vi "host.vi"() -> ()   [LabVIEW 2020]
uses:
  <vilib>/Analysis/baseanly.llb/Real A x B.vi
  <vilib>/Analysis/baseanly.llb/Mean (DBL).vi
  <vilib>/Analysis/Matrix/Numeric/Conversions/Array To Matrix - RA2.vi
  <vilib>/Analysis/Matrix/Numeric/Conversions/Matrix To Array - RM.vi
  <vilib>/Analysis/7linalg.llb/Real Eigenvalues and Vectors.vi
  <vilib>/FPGAPlugInAG/cRIO-9035/niLvFpga_Open_cRIO-9035.vi
  <vilib>/rvi/interface/common/dynamic/niFpgaDynamicAddResources.vi
  <vilib>/Utility/error.llb/Error Cluster From Error Code.vi
  <vilib>/rvi/errors/niLvFpgaAdjustHostInterfaceError.vi
  <vilib>/FPGAPlugInAG/Dynamic/niLvFpga_Run_Dynamic.vi
  <vilib>/FPGAPlugInAG/Dynamic/niLvFpga_Close_Dynamic.vi
  <vilib>/rvi/interface/nirviOpenFPGA/nirviOpenFPGA.xnode
  FPGA Bitfiles/v1.1_FPGATarget_target_IynmV97gzEU.lvbitx
  target.vi
  <vilib>/rvi/interface/nirviMethod/nirviMethod.xnode
  <vilib>/rvi/interface/nirviCloseFPGA/nirviCloseFPGA.xnode
  <vilib>/rvi/errors/niLvFpgaMergeErrorWithErrorCode.vi
  <vilib>/Analysis/Matrix/NI_Matrix.lvlib
  <vilib>/Analysis/NI_AALBase.lvlib
  <vilib>/FPGAPlugInAG/Dynamic/niLvFpga_WriteFifo_Dynamic.vi
  <vilib>/FPGAPlugInAG/Dynamic/niLvFpga_ReadFifo_Dynamic.vi
  <vilib>/Analysis/NI_AALPro.lvlib
panel:
  out "A":dbl[][](array[numeric])
  out "LabVIEW eigvals":dbl[](array[numeric])
  out "FPGA Jacobi eigenvalue":sgl[](array[numeric])
  out "percent error":dbl
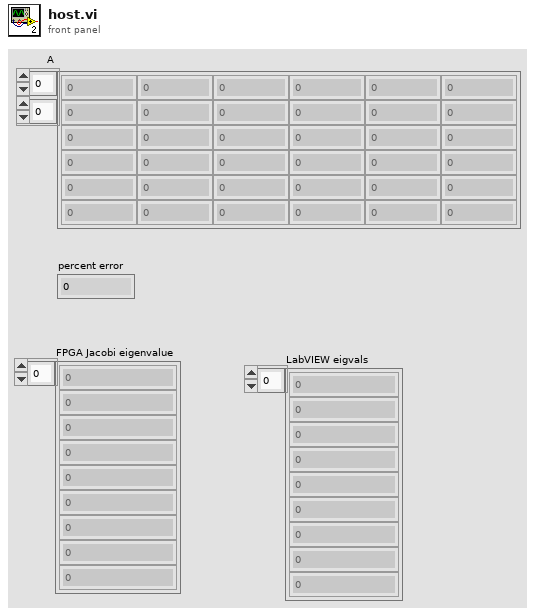
[diagram p1: front panel]
types:
  T1 = typedef "NI_Matrix.lvlib/RealMatrix.ctl" = dbl[][]
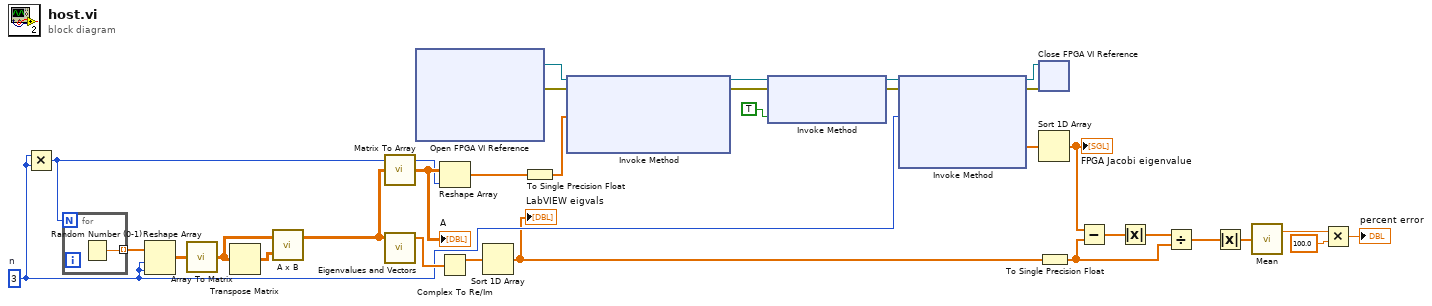
[diagram p0: block diagram]
diagram:
  w19 = 3  # n
  n1 = Multiply(x=w19, y=w19) -> (x*y=w13:i32)
  n2 = for {
    N: w13 -> [_]
    tunnel: [w33] -> w18 mode=indexing
    n3 = Random Number (0-1)() -> (number: 0 to 1=w33:dbl)
  }
  n4 = Reshape Array(w18, w19, w19) -> (w17:dbl[][])
  n5 = call-poly <vilib>:"Array To Matrix.vi"("Real 2D Array"=w17) -> ("Real Matrix"=w16:T1)
  n6 = Transpose Matrix(1:w16) -> (0:w15:T1)
  n7 = call-poly <vilib>:"A x B.vi"("B"=w15, "A"=w16) -> ("A x B"=w24:T1)  [unwired: 1 out]
  n8 = call-poly <vilib>:"Matrix To Array.vi"("Real Matrix"=w24) -> ("Real 2D Array"=w22:dbl[][])
  "A" <- w22
  n9 = call-poly <vilib>:"Eigenvalues and Vectors.vi"("Input Matrix"=w24) -> ("Eigenvalues"=w25:cdb[])  [unwired: 2 in, 2 out]
  n10 = xnode "Open FPGA VI Reference"() -> ("FPGA VI Reference Out"=w31:refnum<k20>, "error out"=w30:errorcluster)  [unwired: 2 in]
  n11 = Reshape Array(w22, w13) -> (w14:dbl[])
  n12 = Complex To Re/Im(x + iy=w25) -> (x=w23:dbl[])  [unwired: 1 out]
  n13 = Sort 1D Array(array=w23) -> (sorted array=w12:dbl[])
  "LabVIEW eigvals" <- w12
  n14 = To Single Precision Float(number=w14) -> (single precision float=w21:sgl[])
  n15 = xnode "Invoke Method"("FPGA VI Reference In"=w31, "error in"=w30, "Data"=w21) -> ("FPGA VI Reference Out"=w27:refnum<k20>, "error out"=w26:errorcluster)  [unwired: 1 in, 1 out]
  n16 = xnode "Invoke Method"("FPGA VI Reference In"=w27, "error in"=w26, "Wait Until Done (F)"=TRUE) -> ("FPGA VI Reference Out"=w29:refnum<k20>, "error out"=w28:errorcluster)
  n17 = xnode "Invoke Method"("FPGA VI Reference In"=w29, "error in"=w28, "Number of Elements"=w19) -> ("FPGA VI Reference Out"=w2:refnum<k20>, "error out"=w1:errorcluster, "Data"=w20:sgl[])  [unwired: 1 in, 1 out]
  n18 = xnode "Close FPGA VI Reference"("FPGA VI Reference In"=w2, "error in"=w1) -> ()  [unwired: 1 out]
  n19 = Sort 1D Array(array=w20) -> (sorted array=w11:sgl[])
  "FPGA Jacobi eigenvalue" <- w11
  n20 = To Single Precision Float(number=w12) -> (single precision float=w8:sgl[])
  n21 = Subtract(x=w11, y=w8) -> (x-y=w10:sgl[])
  n22 = Absolute Value(x=w10) -> (abs(x)=w9:sgl[])
  n23 = Divide(x=w9, y=w8) -> (x/y=w7:sgl[])
  n24 = Absolute Value(x=w7) -> (abs(x)=w6:sgl[])
  n25 = call-poly <vilib>:"Mean.vi"("X"=w6) -> ("mean"=w5:dbl)  [unwired: 1 out]
  n26 = Multiply(x=w5, y=100.0) -> (x*y=→"percent error":dbl)
